vi "Format Gas Params Refactored.vi"() -> ()   [LabVIEW 2012]
panel:
  in  "错误输入":cluster{"状态":bool, "代码":i32, "源":string}
  out "错误输出":cluster{"状态":bool, "代码":i32, "源":string}
  out "结果":string
  in  "气体参数名称":string[](array[string])=["温度", "气压", "湿度", "体积", "密度"]
  in  "气体参数值":dbl[](array[numeric])=[1.0, 2.0, 3.0, 4.0, 5.0]
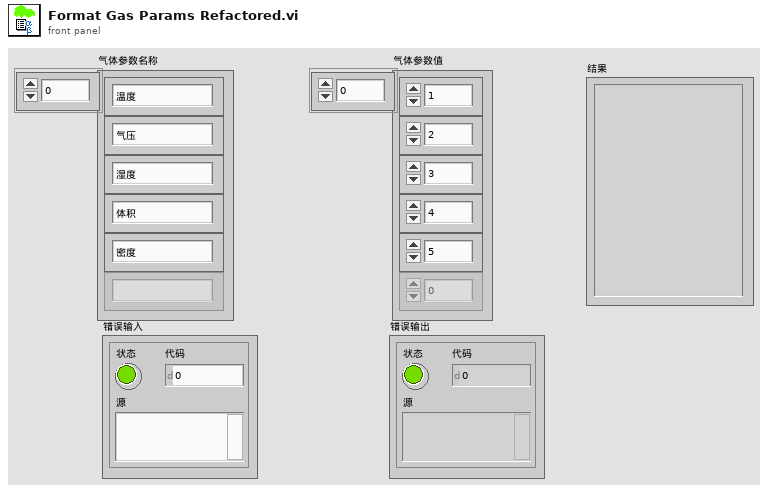
[diagram p1: front panel]
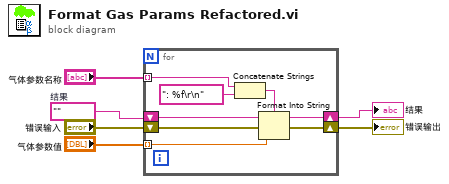
[diagram p0: block diagram]
diagram:
  w3 = ""  # 结果
  n1 = for {
    tunnel: "气体参数值" -> [w7] mode=indexing
    shift-right: [w9] -> w4
    shift-left: w3 -> [w10]
    tunnel: "气体参数名称" -> [w14] mode=indexing
    shift-right: [w11] -> w2
    shift-left: "错误输入" -> [w8]
    n2 = Concatenate Strings ("连接字符串")(w14, ": %f\r\n" ("字符串")) -> (w12:string)
    n3 = Format Into String ("格式化写入字符串")(format string=w12, initial string=w10, error in=w8, w7) -> (resulting string=w9:string, error out=w11:errorcluster)
  }
  "结果" <- w4
  "错误输出" <- w2
